vi "io.vi"(4 "tick":bool, 5 "Control":T5, 6 "r_all":bool, 7 "WR":T4, 8 "RD":T4, 9 "from":T3) -> (0 "flag_reg":T1, 1 "reg_acc":T2, 2 "reg_b":T2, 3 "reg_a":T2)   [LabVIEW 2013]
panel:
  # "R1"
  # "R1"
  # "R1"
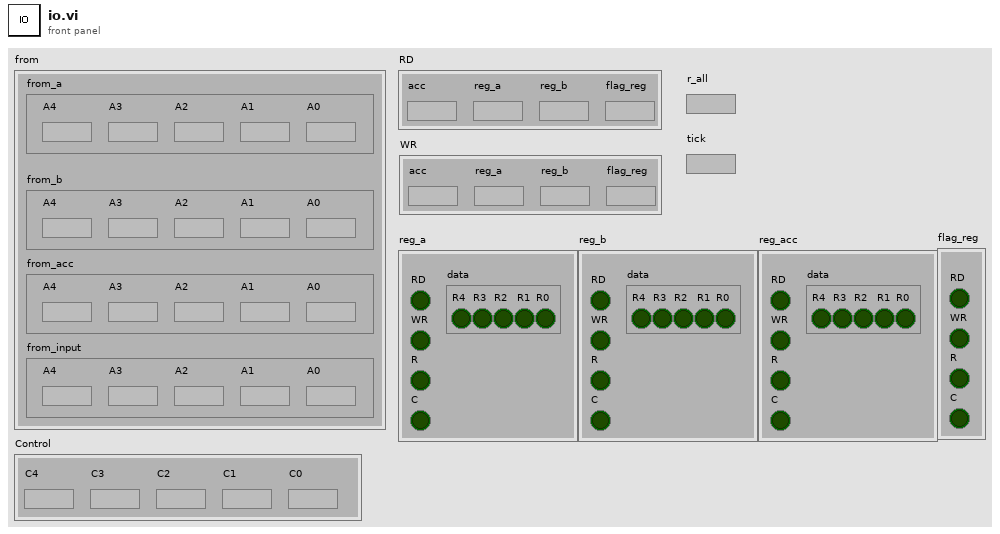
[diagram p1: front panel]
types:
  T1 = cluster{"RD":bool, "WR":bool, "R":bool, "C":bool}
  T2 = cluster{"RD":bool, "WR":bool, "R":bool, "C":bool, "data":cluster{"R4":bool, "R3":bool, "R2":bool, bool, "R0":bool}}
  T3 = cluster{"from_a":cluster{"A4":bool, "A3":bool, "A2":bool, "A1":bool, "A0":bool}, "from_b":cluster{"A4":bool, "A3":bool, "A2":bool, "A1":bool, "A0":bool}, "from_acc":cluster{"A4":bool, "A3":bool, "A2":bool, "A1":bool, "A0":bool}, "from_input":cluster{"A4":bool, "A3":bool, "A2":bool, "A1":bool, "A0":bool}}
  T4 = cluster{"acc":bool, "reg_a":bool, "reg_b":bool, "flag_reg":bool}
  T5 = cluster{"C4":bool, "C3":bool, "C2":bool, "C1":bool, "C0":bool}
  T6 = cluster{"A4":bool, "A3":bool, "A2":bool, "A1":bool, "A0":bool}
  T7 = cluster{bool, "reg_a":bool, "r_all":bool, "tick":bool, cluster{"A4":bool, "A3":bool, "A2":bool, "A1":bool, "A0":bool}}
  T8 = cluster{bool, bool, "r_all":bool, "tick":bool, cluster{"A4":bool, "A3":bool, "A2":bool, "A1":bool, "A0":bool}}
  T9 = cluster{bool, "reg_b":bool, "r_all":bool, "tick":bool, cluster{"A4":bool, "A3":bool, "A2":bool, "A1":bool, "A0":bool}}
  T10 = cluster{bool, "flag_reg":bool, "r_all":bool, "tick":bool}
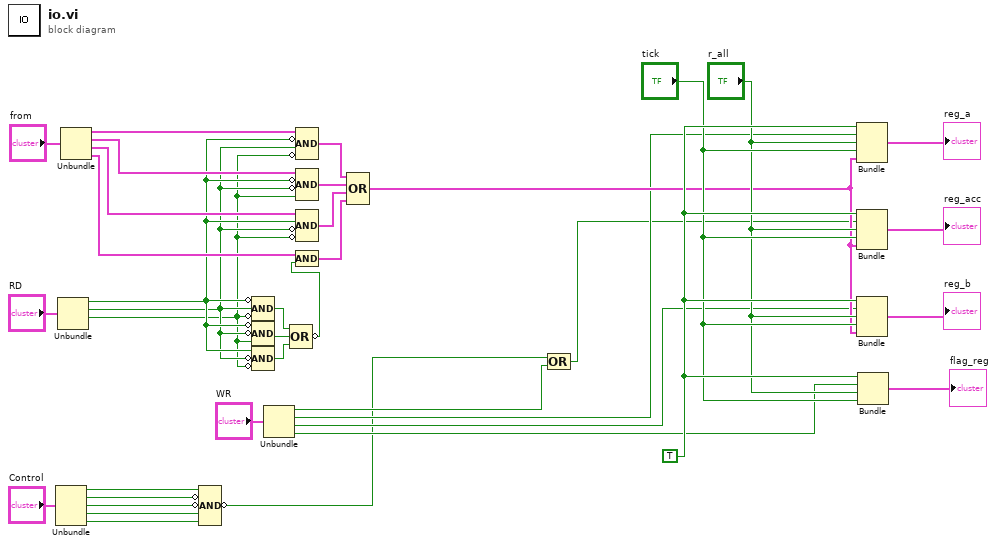
[diagram p0: block diagram]
diagram:
  w10 = TRUE
  n1 = Unbundle("Control") -> ("C4"=w35:bool, "C3"=w34:bool, "C2"=w33:bool, "C1"=w32:bool, "C0"=w31:bool)
  n2 = Unbundle("RD") -> ("acc"=w14:bool, "reg_a"=w13:bool, "reg_b"=w12:bool)  [unwired: 1 out]
  n3 = Unbundle("from") -> ("from_a"=w22:T6, "from_b"=w19:T6, "from_acc"=w20:T6, "from_input"=w21:T6)
  n4 = Compound Arithmetic op=AND(w35, invert w34, invert w33, w32, w31) -> (invert w1:bool)
  n5 = Compound Arithmetic op=AND(invert w14, w13, invert w12) -> (w18:bool)
  n6 = Compound Arithmetic op=AND(invert w14, invert w13, w12) -> (w17:bool)
  n7 = Compound Arithmetic op=AND(w14, invert w13, invert w12) -> (w16:bool)
  n8 = Unbundle("WR") -> ("acc"=w2:bool, "reg_a"=w6:bool, "reg_b"=w5:bool, "flag_reg"=w4:bool)
  n9 = Compound Arithmetic op=OR(w18, w17, w16) -> (invert w15:bool)
  n10 = Compound Arithmetic op=AND(w22, invert w14, w13, invert w12) -> (w26:T6)
  n11 = Compound Arithmetic op=AND(w19, invert w14, invert w13, w12) -> (w23:T6)
  n12 = Compound Arithmetic op=AND(w20, w14, invert w13, invert w12) -> (w24:T6)
  n13 = Compound Arithmetic op=AND(w21, w15) -> (w25:T6)
  n14 = Compound Arithmetic op=OR(w26, w23, w24, w25) -> (w7:T6)
  n15 = Compound Arithmetic op=OR(w1, w2) -> (w3:bool)
  n16 = Bundle(w10, "reg_a"=w6, "r_all"="r_all", "tick"="tick", w7) -> (→"reg_a":T7)  [unwired: 1 in]
  n17 = Bundle(w10, w3, "r_all"="r_all", "tick"="tick", w7) -> (→"reg_acc":T8)  [unwired: 1 in]
  n18 = Bundle(w10, "reg_b"=w5, "r_all"="r_all", "tick"="tick", w7) -> (→"reg_b":T9)  [unwired: 1 in]
  n19 = Bundle(w10, "flag_reg"=w4, "r_all"="r_all", "tick"="tick") -> (→"flag_reg":T10)  [unwired: 1 in]
